vi "cRIO Led Ansteuerung.vi"(8 "error in (no error)":errorcluster) -> (0 "error out":errorcluster caption="Fehler (Ausgang)")   [LabVIEW 2020, in "Allgemein.lvlib"]
uses:
  Allgemein.lvlib
  <vilib>/NI_Real-Time Target Support.lvlib
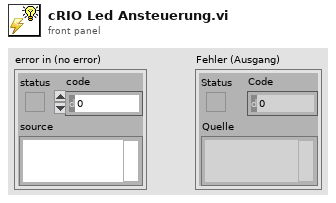
[diagram p1: front panel]
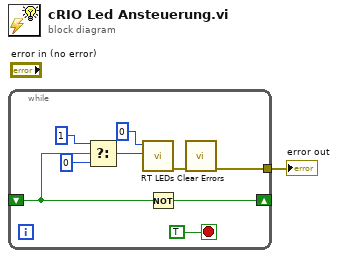
[diagram p0: block diagram]
diagram:
  n1 = while {
    shift-right: [w6] -> _
    shift-left: _ -> [w5]
    tunnel: [w2] -> w1
    stop <- TRUE stop-if-true
    n2 = Select(t=1 ("State"), s=w5, f=0) -> (s? t:f=w7:i32)
    n3 = call <vilib>:"RT LEDs.vi"("State"=w7, "LED Num"=0) -> ("error out"=w10:errorcluster)  [unwired: 4 in, 1 out]
    n4 = Not(x=w5) -> (.not. x?=w6:bool)
    n5 = call <vilib>:"Clear Errors.vi"("error in (no error)"=w10) -> ("error out"=w2:errorcluster)  [unwired: 5 in, 1 out]
  }
  "error out" <- w1
